vi "Trajectory_Execution_Set_Auto.vi"(11 "Ramsete AUTO":bool) -> ()   [LabVIEW 2019]
uses:
  Trajectory_Execution_Globals.vi
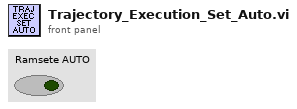
[diagram p1: front panel]
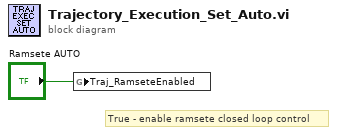
[diagram p0: block diagram]
diagram:
  # "True - enable ramsete closed loop control"
  n1 = global write "Trajectory_Execution_Globals.vi" "Traj_RamseteEnabled"("Ramsete AUTO") -> ()
